vi "Exam 1 Question 1.vi"() -> ()   [LabVIEW 2016]
panel:
  out "Result":dbl
  in  "Operation":string
  in  "Opperand 2":dbl
  in  "Opperand 1":dbl
  # "* = multiplication \n+ = addition \n- = subtraction \n/ = division"
  # "This is a string"
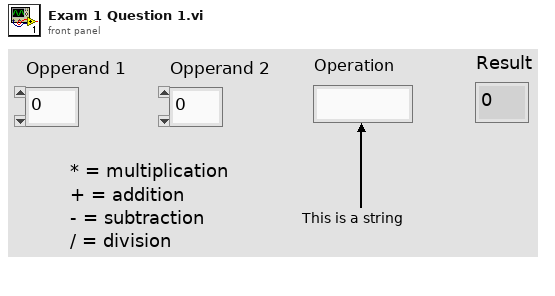
[diagram p1: front panel]
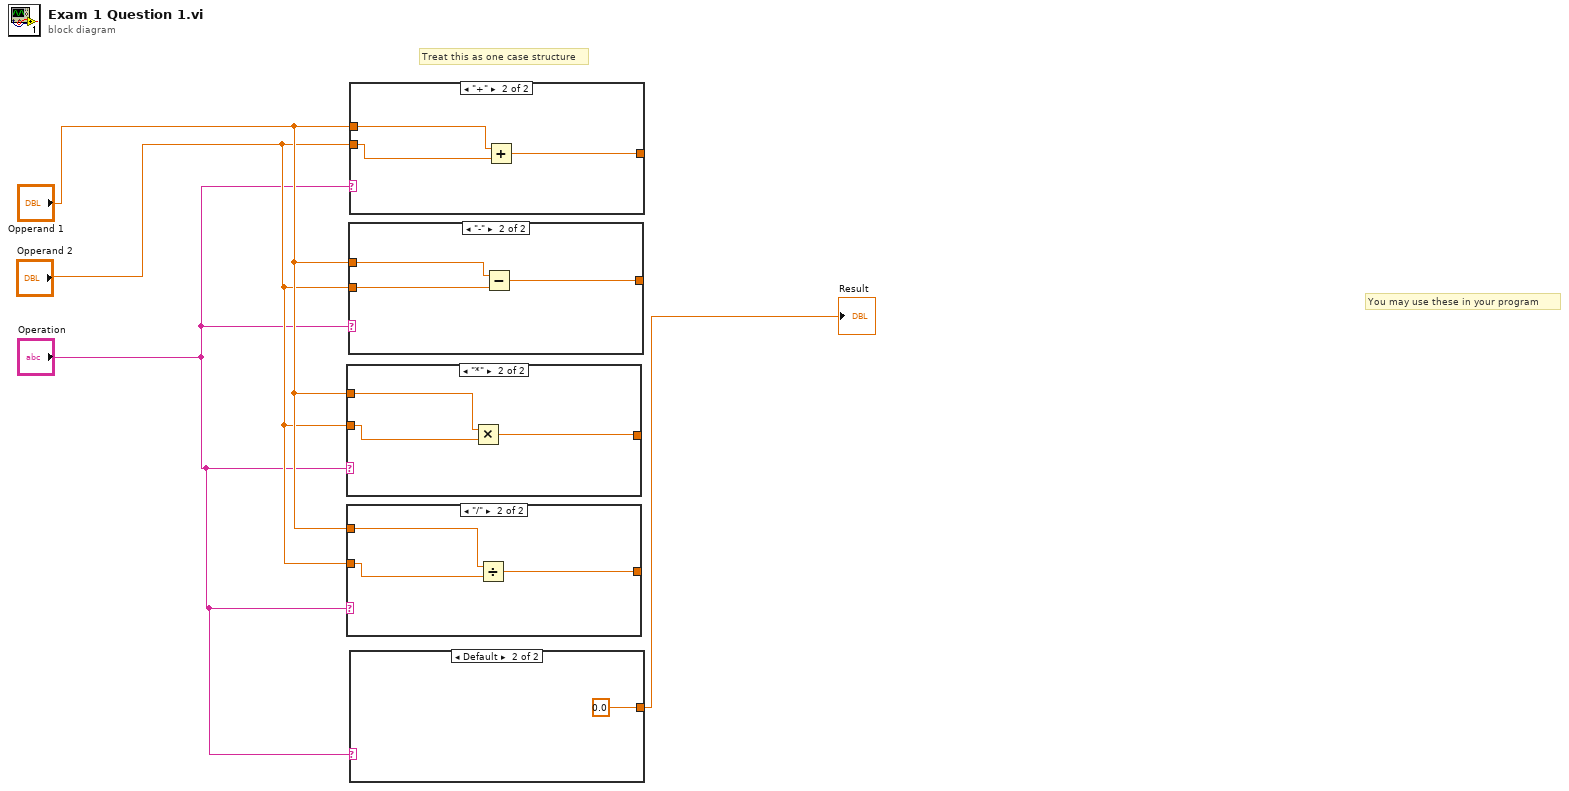
[diagram p0: block diagram]
diagram:
  # "You may use these in your program"
  # "Treat this as one case structure"
  n1 = case shown="\"*\"" "Operation" {
    tunnel: "Opperand 1" -> [_ w6]
    tunnel: "Opperand 2" -> [_ w5]
    tunnel: [_ w7] -> _
    frame "False", Default {
    }
    frame "*" {
      n2 = Multiply(x=w6, y=w5) -> (x*y=w7:dbl)
    }
  }
  n3 = case shown="\"/\"" "Operation" {
    tunnel: "Opperand 1" -> [_ w9]
    tunnel: "Opperand 2" -> [_ w8]
    tunnel: [_ w10] -> _
    frame "False", Default {
    }
    frame "/" {
      n4 = Divide(x=w9, y=w8) -> (x/y=w10:dbl)
    }
  }
  n5 = case shown="\"-\"" "Operation" {
    tunnel: "Opperand 1" -> [_ w12]
    tunnel: "Opperand 2" -> [_ w11]
    tunnel: [_ w13] -> _
    frame "False", Default {
    }
    frame "-" {
      n6 = Subtract(x=w12, y=w11) -> (x-y=w13:dbl)
    }
  }
  n7 = case shown="\"+\"" "Operation" {
    tunnel: "Opperand 1" -> [_ w15]
    tunnel: "Opperand 2" -> [_ w14]
    tunnel: [_ w16] -> _
    frame "False", Default {
    }
    frame "+" {
      n8 = Add(x=w15, y=w14) -> (x+y=w16:dbl)
    }
  }
  n9 = case shown="Default" "Operation" {
    tunnel: [_ 0.0] -> w2
    frame "False" {
    }
    frame Default {
    }
  }
  "Result" <- w2
